vi "new_issue_partial.vi"(6 "name":string, 8 "number":string, 9 "small cover url":string, 10 "url":string, 11 "id":string) -> (3 "issue_class out":refnum<class "issue_class.lvclass">)   [LabVIEW 2024, in "issue_class.lvclass"]
uses:
  issue_class.lvclass
  issue_class.lvclass/issue_class.ctl
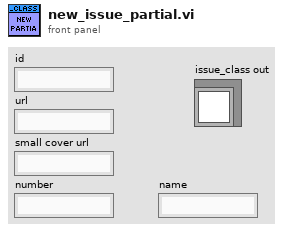
[diagram p1: front panel]
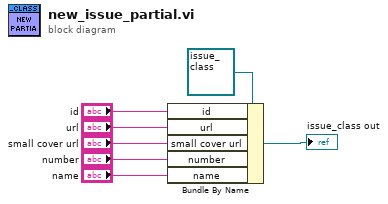
[diagram p0: block diagram]
diagram:
  n1 = Bundle By Name(cluster=refnum<class "issue_class.lvclass"> refnum ("issue_class in"), "id"="id", "url"="url", "small cover url"="small cover url", "number"="number", "name"="name") -> (→"issue_class out":refnum<class "issue_class.lvclass">)
